vi "Verify Callback Path.vi"(7 "Parent VI Ref":refnum<vi>, 8 "error in (no error)":errorcluster, 11 "Saved Callback Path":path) -> (0 "error out":errorcluster, 3 "Valid Path out":string)   [LabVIEW 2021]
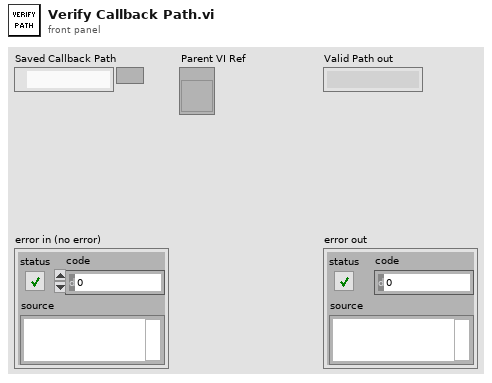
[diagram p1: front panel]
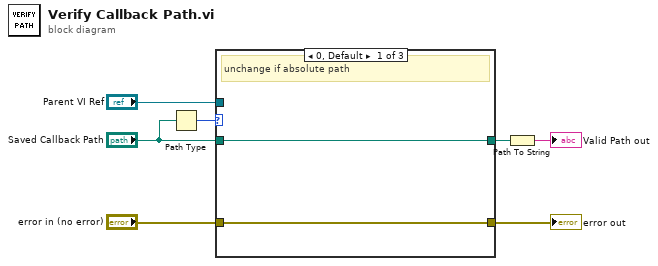
[diagram p0: block diagram]
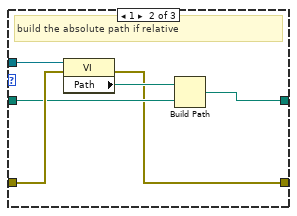
[diagram p2: hidden frame]
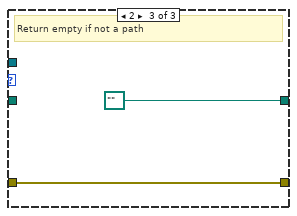
[diagram p3: hidden frame]
diagram:
  n1 = Path Type(1:"Saved Callback Path") -> (0:w4:i16)
  n2 = case shown="0, Default" w4 {
    tunnel: [w8 w11 path "" ("Saved Path")] -> w1
    tunnel: "Saved Callback Path" -> [w8 w12 _]
    tunnel: "Parent VI Ref" -> [_ w14 _]
    tunnel: "error in (no error)" -> [w9 w13 w16]
    tunnel: [w9 w10 w16] -> w7
    frame 0, Default {
      # "unchange if absolute path"
    }
    frame 1 {
      # "build the absolute path if relative"
      n3 = property class="VI"(reference=w14, error in=w13) -> (error out=w10:errorcluster, "Path"=w15:path)  [unwired: 1 out]
      n4 = Build Path(base path=w15, name or relative path=w12) -> (appended path=w11:path)
    }
    frame 2 {
      # "Return empty if not a path"
    }
  }
  "error out" <- w7
  n5 = Path To String(path=w1) -> (string=→"Valid Path out":string)
